vi "mislanius_time_add_all.vi"(0 "Select Product":string, 1 "Cluster":T2={"connection reference"=refnum, "Net Avai time (Min)"=0, "pLAN dATE datA"=[], "Data by plan date, shift, product"=[], "BreakDownd Data"=[], "Raw rejection Data"=[], "mislanius times shift 1"={"Lunch Time From"=timestamp(0 s since 1904-01-01), "Lunch Time To"=timestamp(0 s since 1904-01-01), "Tea Time From"=timestamp(0 s since 1904-01-01), "Tea Time To"=timestamp(0 s since 1904-01-01), "Clean Time From"=timestamp(0 s since 1904-01-01), "Clean Time To"=timestamp(0 s since 1904-01-01), "Meeting Time From"=timestamp(0 s since 1904-01-01), "Meeting Time To"=timestamp(0 s since 1904-01-01), "Dev/Other Time From"=timestamp(0 s since 1904-01-01), "Dev/Other Time To"=timestamp(0 s since 1904-01-01), "Meeting"=FALSE, "Dev/Other"=TRUE}, "mislanius times shift 2"={"Lunch Time From"=timestamp(0 s since 1904-01-01), "Lunch Time To"=timestamp(0 s since 1904-01-01), "Tea Time From"=timestamp(0 s since 1904-01-01), "Tea Time To"=timestamp(0 s since 1904-01-01), "Clean Time From"=timestamp(0 s since 1904-01-01), "Clean Time To"=timestamp(0 s since 1904-01-01), "Meeting Time From"=timestamp(0 s since 1904-01-01), "Meeting Time To"=timestamp(0 s since 1904-01-01), "Dev/Other Time From"=timestamp(0 s since 1904-01-01), "Dev/Other Time To"=timestamp(0 s since 1904-01-01), "Meeting"=FALSE, "Dev/Other"=TRUE}} {"mislanius times shift 2"."Lunch Time From" format="%<%.X %x>T"; "mislanius times shift 2"."Lunch Time To" format="%<%.X %x>T"; "mislanius times shift 2"."Tea Time From" format="%<%.X %x>T"; "mislanius times shift 2"."Tea Time To" format="%<%.X %x>T"; "mislanius times shift 2"."Clean Time From" format="%<%.X %x>T"; "mislanius times shift 2"."Clean Time To" format="%<%.X %x>T"; "mislanius times shift 2"."Meeting Time From" format="%<%.X %x>T"; "mislanius times shift 2"."Meeting Time To" format="%<%.X %x>T"; "mislanius times shift 2"."Dev/Other Time From" format="%<%.X %x>T"; "mislanius times shift 2"."Dev/Other Time To" format="%<%.X %x>T"; "mislanius times shift 1"."Lunch Time From" format="%<%.X %x>T"; "mislanius times shift 1"."Lunch Time To" format="%<%.X %x>T"; "mislanius times shift 1"."Tea Time From" format="%<%.X %x>T"; "mislanius times shift 1"."Tea Time To" format="%<%.X %x>T"; "mislanius times shift 1"."Clean Time From" format="%<%.X %x>T"; "mislanius times shift 1"."Clean Time To" format="%<%.X %x>T"; "mislanius times shift 1"."Meeting Time From" format="%<%.X %x>T"; "mislanius times shift 1"."Meeting Time To" format="%<%.X %x>T"; "mislanius times shift 1"."Dev/Other Time From" format="%<%.X %x>T"; "mislanius times shift 1"."Dev/Other Time To" format="%<%.X %x>T"}, 2 "error in (no error)":errorcluster, 3 "Date":timestamp, 8 "Shift":string(combo)="2") -> (6 "AT min":i32, 10 "Split DT time":u32[](array[numeric]), 12 "Only select product and date and shift data":string[][](array[string]), 15 "1st and last cycle time stamp":timestamp[](array[timestamp]), 16 "error out":errorcluster, 17 "Net Available Time":u32, 18 "output cluster":T1, 19 "Total mis time":i32)   [LabVIEW 2017]
uses:
  Controls/OE_screen_cluster.ctl
  <vilib>/addons/database/Connection.llb/Conn ObjectReference.ctl
  <userlib>/_OpenG.lib/array/array.llb/Remove Duplicates from 1D Array (String)__ogtk.vi
  <userlib>/_OpenG.lib/array/array.llb/Search 1D Array (String)__ogtk.vi
  <userlib>/_OpenG.lib/array/array.llb/Remove Duplicates from 1D Array (I32)__ogtk.vi
  <vilib>/addons/database/NI_Database_API.lvlib
panel:
  out "Array":string[](array[string])
  out "x-1 3":timestamp[](array[timestamp])
  out "Array 2":timestamp[](array[timestamp])
  out "indices of removed elements":i32[](array[numeric])
  out "Only rejected- select product and date and shift data":string[][](array[string])
  out "Parts per hour":i32
  out "Lunch time 3":i32
  out "tea time 3":i32
  out "clean time 3":i32
  out "meeting time 3":i32
  out "Dev/other time 3":i32
  out "Lunch time 2":i32
  out "tea time 2":i32
  out "clean time 2":i32
  out "meeting time 2":i32
  out "Dev/other time 2":i32
  out "Dev/other time":i32
  out "meeting time":i32
  out "clean time":i32
  out "tea time":i32
  out "Lunch time":i32
  out "In Range? 5":bool
  out "In Range? 4":bool
  out "In Range? 3":bool
  out "In Range? 2":bool
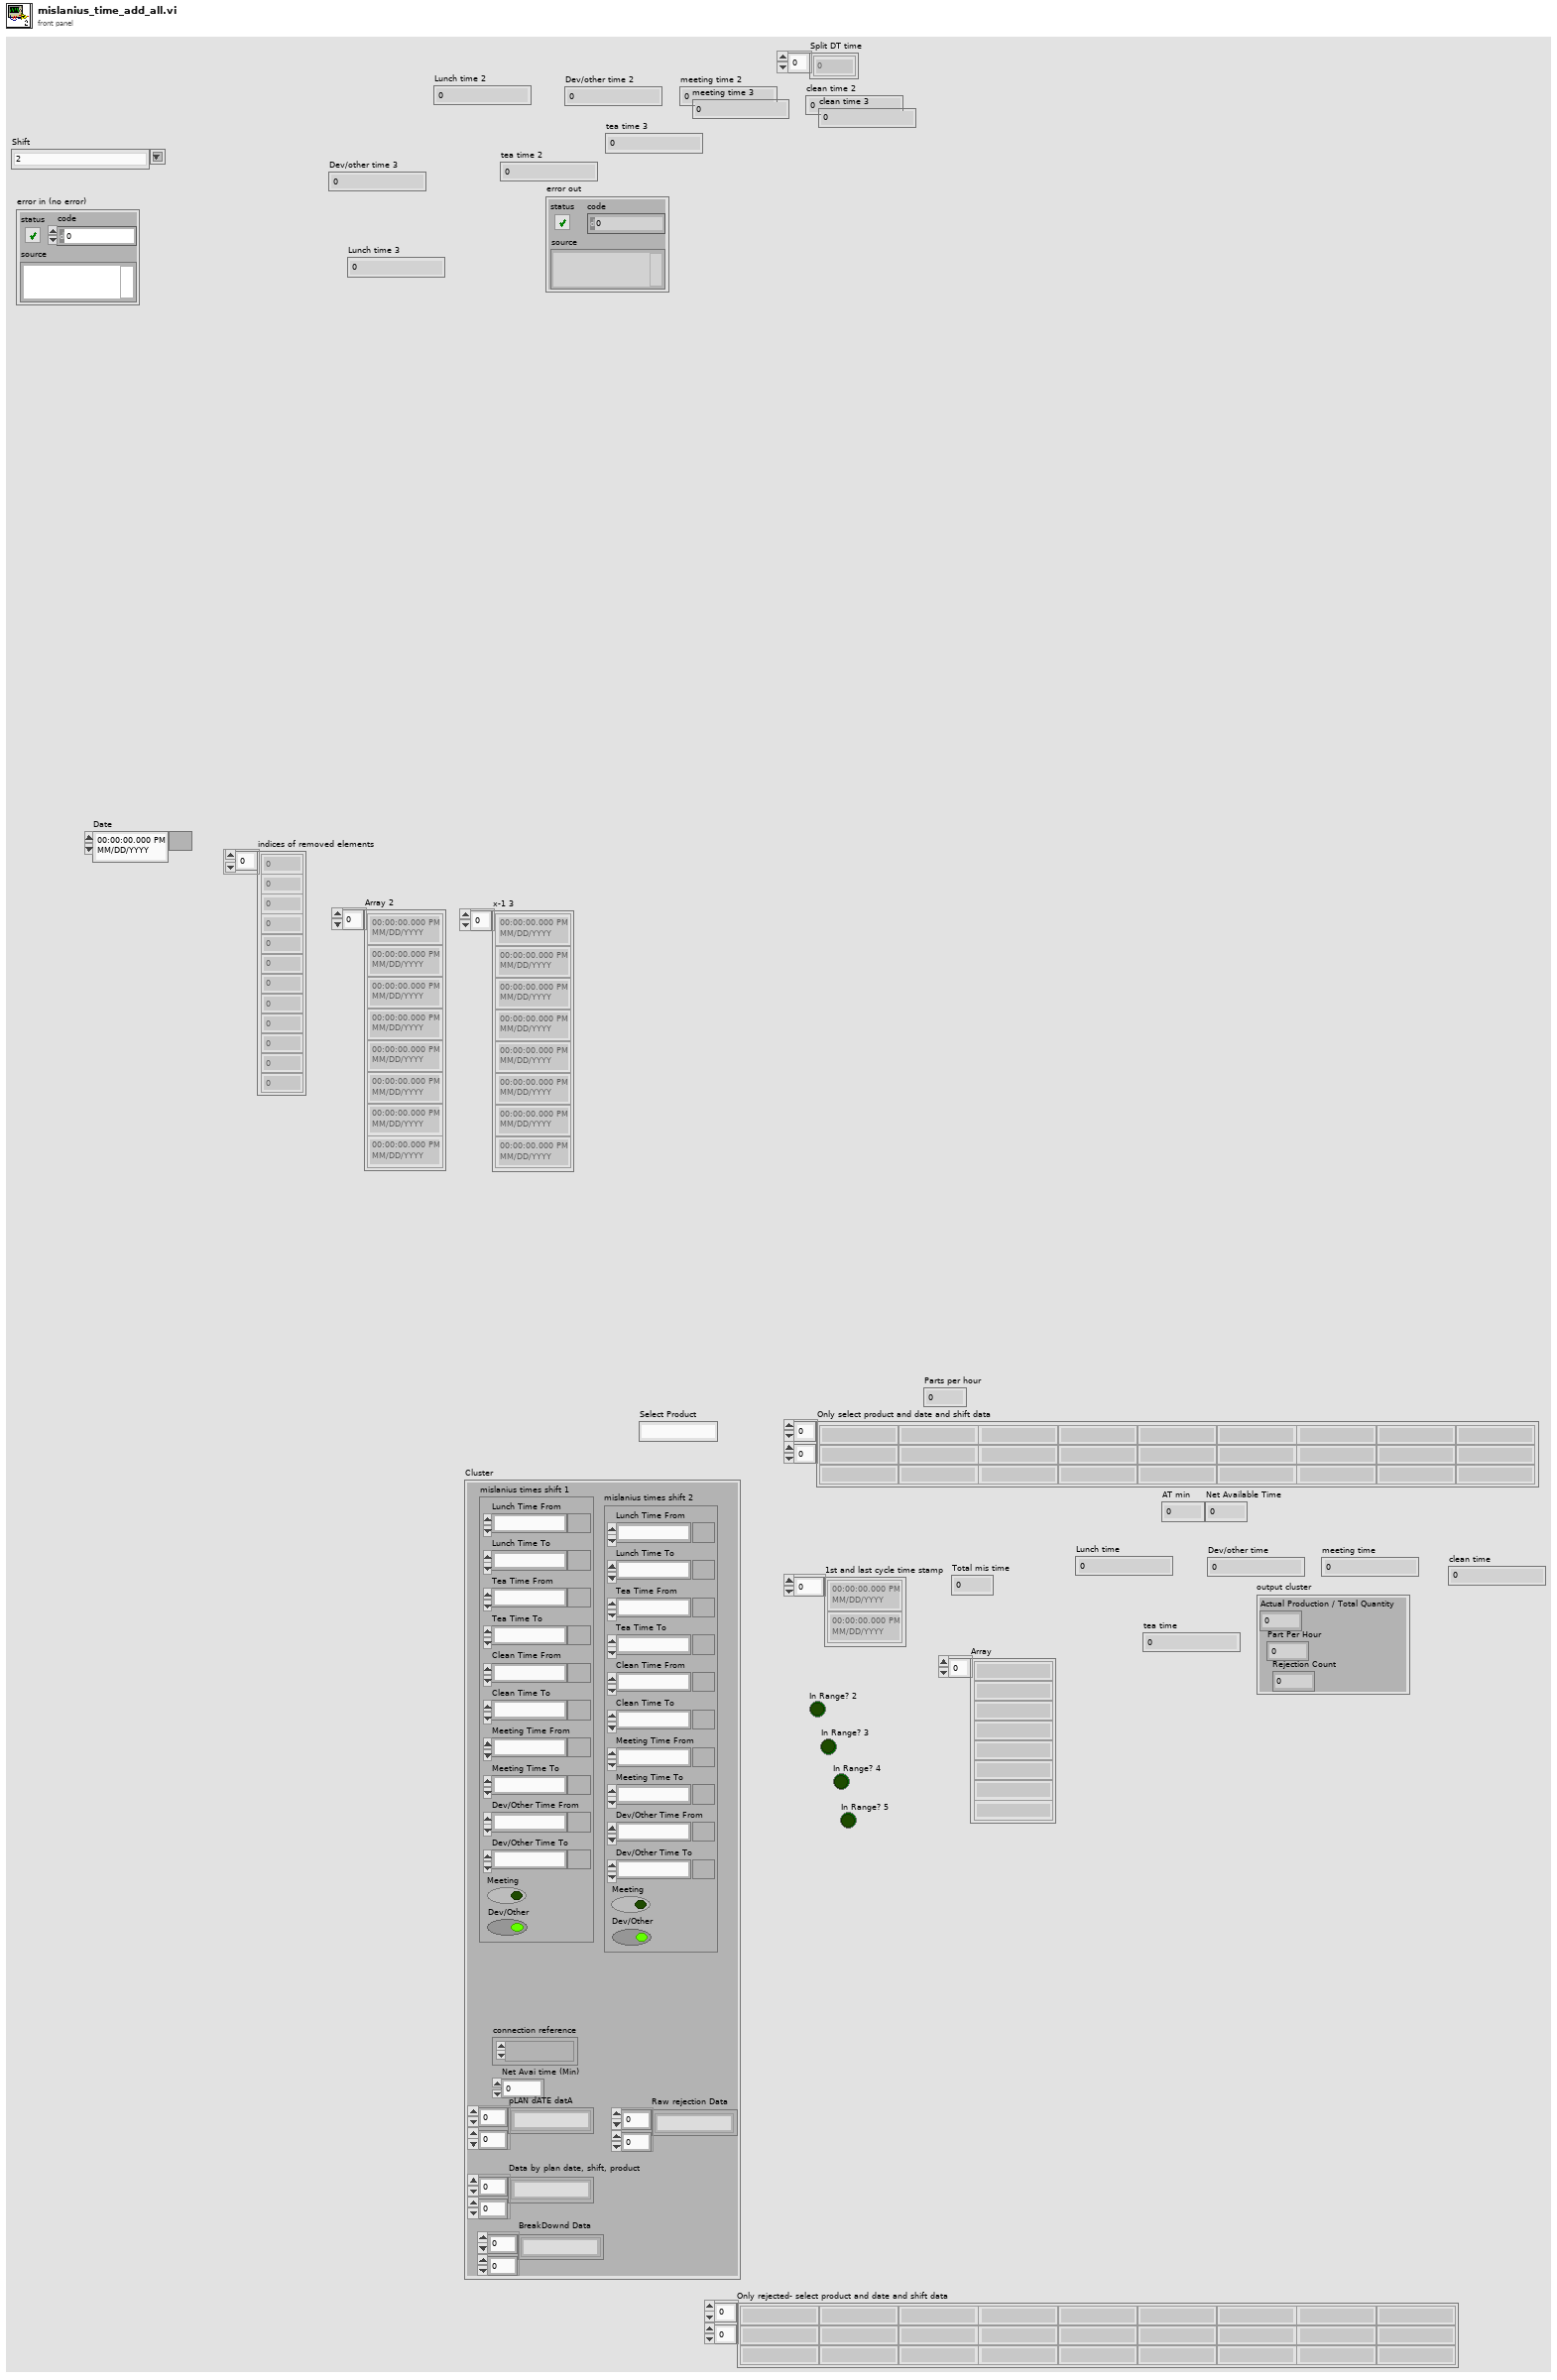
[diagram p1: front panel]
types:
  T1 = cluster{"Actual Production / Total Quantity":u32, "Part Per Hour":i16, "Rejection Count":u32}
  T2 = typedef "OE_screen_cluster.ctl" = cluster{"connection reference":T3, "Net Avai time (Min)":i32, "pLAN dATE datA":string[][], "Data by plan date, shift, product":string[][], "BreakDownd Data":string[][], "Raw rejection Data":string[][], "mislanius times shift 1":cluster{"Lunch Time From":timestamp, "Lunch Time To":timestamp, "Tea Time From":timestamp, "Tea Time To":timestamp, "Clean Time From":timestamp, "Clean Time To":timestamp, "Meeting Time From":timestamp, "Meeting Time To":timestamp, "Dev/Other Time From":timestamp, "Dev/Other Time To":timestamp, "Meeting":bool, "Dev/Other":bool}, "mislanius times shift 2":cluster{"Lunch Time From":timestamp, "Lunch Time To":timestamp, "Tea Time From":timestamp, "Tea Time To":timestamp, "Clean Time From":timestamp, "Clean Time To":timestamp, "Meeting Time From":timestamp, "Meeting Time To":timestamp, "Dev/Other Time From":timestamp, "Dev/Other Time To":timestamp, "Meeting":bool, "Dev/Other":bool}}
  T3 = typedef "NI_Database_API.lvlib/Conn ObjectReference.ctl" = refnum<k1>
  T4 = typedef "LVDateTimeRec.ctl" = cluster{"fractional second":dbl, "second":i32, "minute":i32, "hour":i32, "day of month":i32, "month":i32, "year":i32, "day of week":i32, "day of year":i32, "DST":i32}
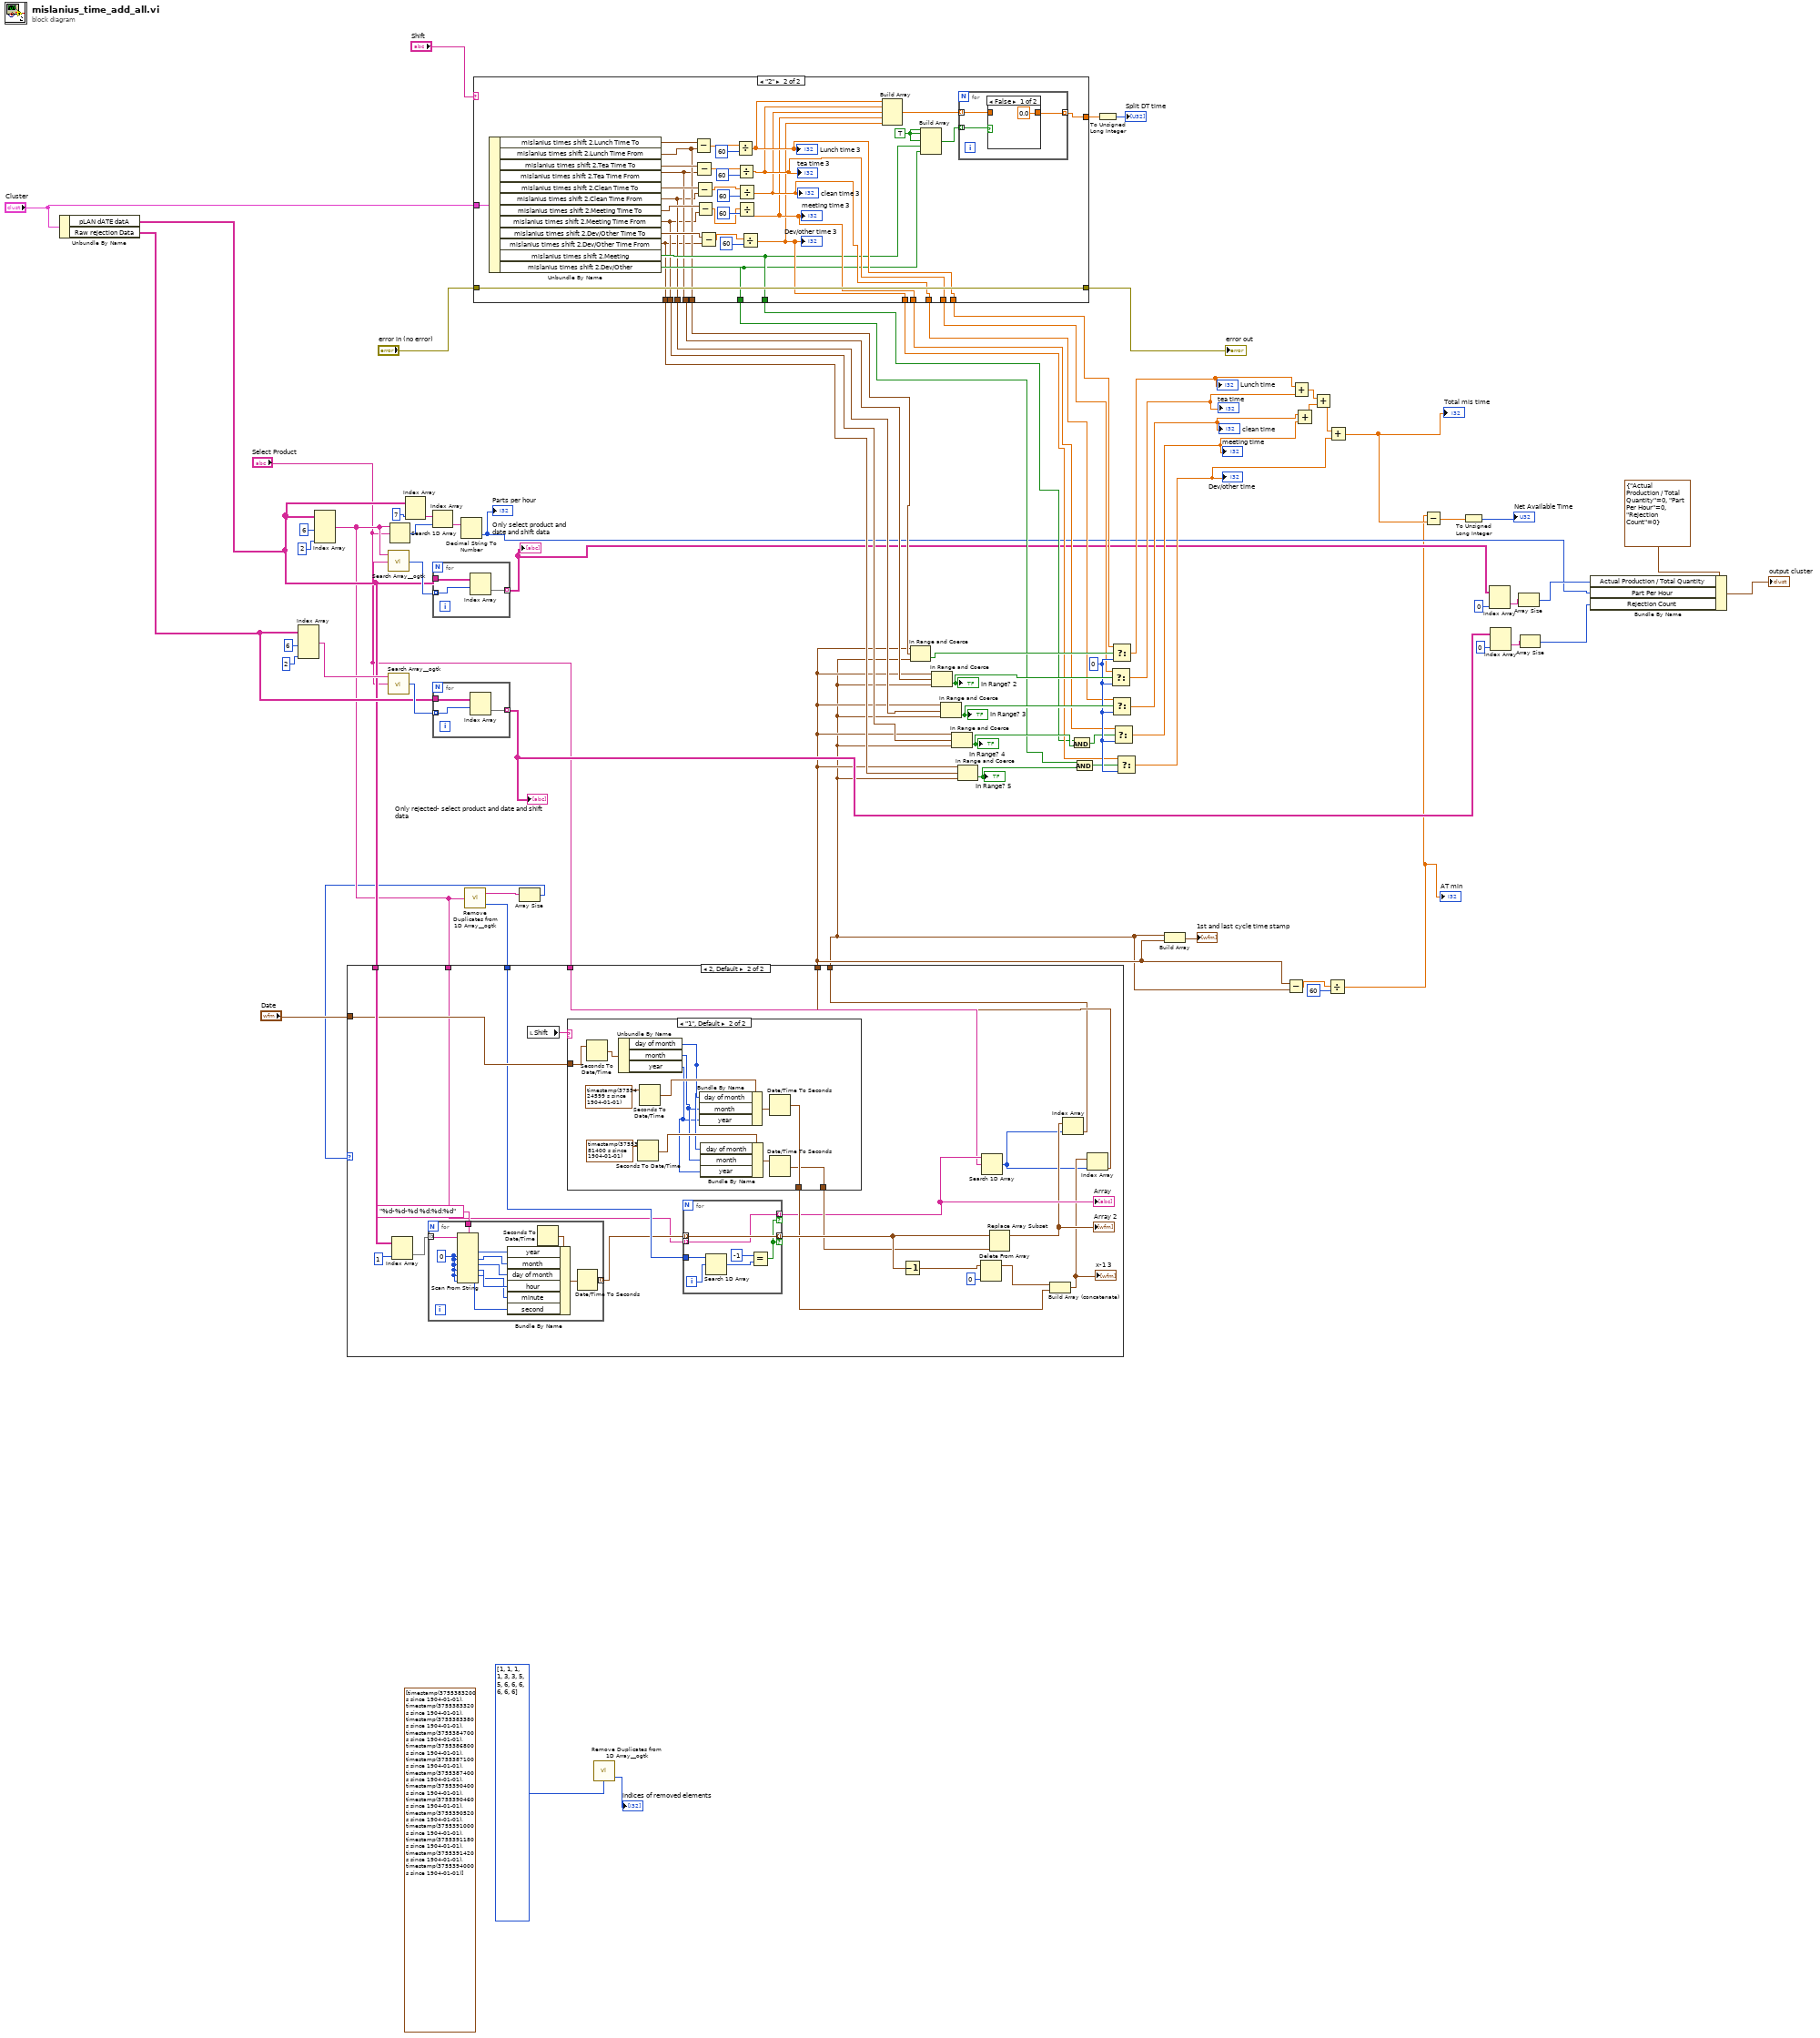
[diagram p0: block diagram]
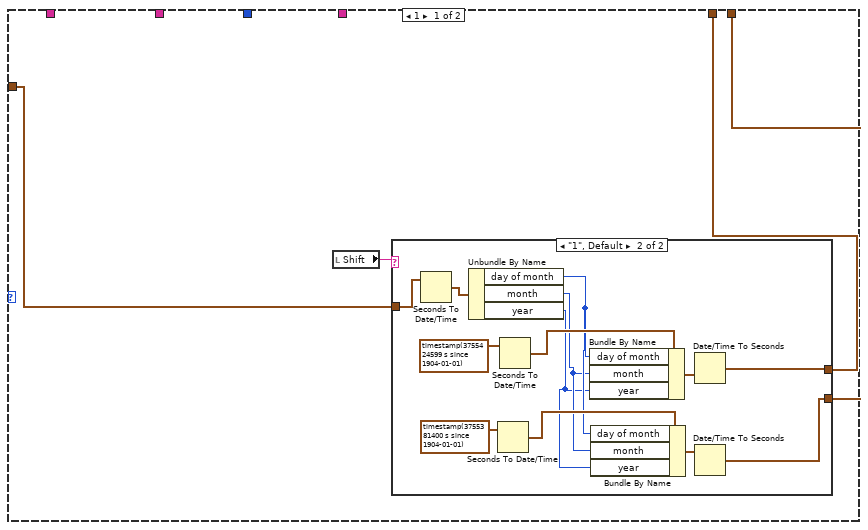
[diagram p2: hidden frame]
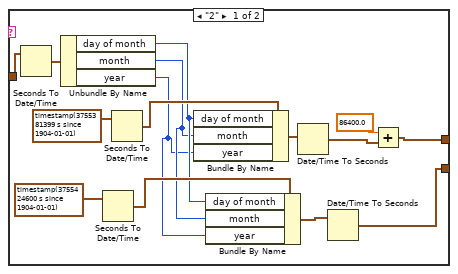
[diagram p3: hidden frame]
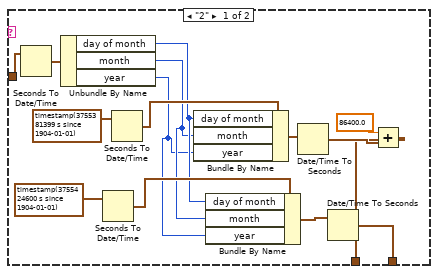
[diagram p4: hidden frame]
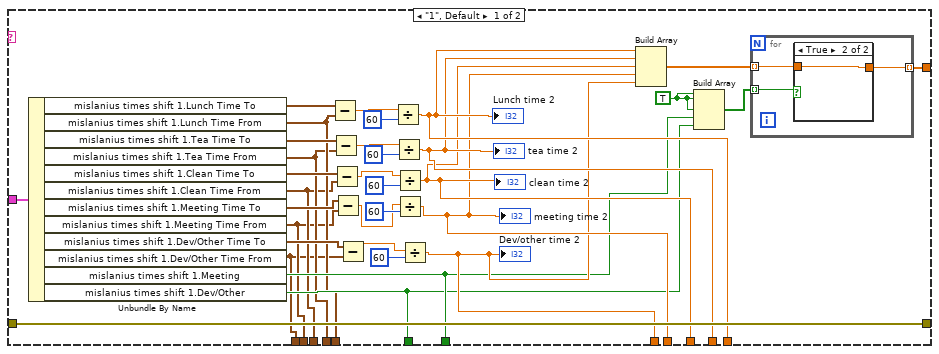
[diagram p5: hidden frame]
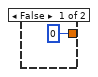
[diagram p6: hidden frame]
diagram:
  (unwired) timestamp[] [timestamp(3755383200 s since 1904-01-01), timestamp(3755383320 s since 1904-01-01), timestamp(3755383380 s since 1904-01-01), timestamp(3755384700 s since 1904-01-01), timestamp(3755386800 s since 1904-01-01), timestamp(3755387100 s since 1904-01-01), timestamp(3755387400 s since 1904-01-01), timestamp(3755390400 s since 1904-01-01), timestamp(3755390460 s since 1904-01-01), timestamp(3755390520 s since 1904-01-01), timestamp(3755391000 s since 1904-01-01), timestamp(3755391180 s since 1904-01-01), timestamp(3755391420 s since 1904-01-01), timestamp(3755394000 s since 1904-01-01)]
  w66 = 0
  n1 = Unbundle By Name("Cluster") -> ("pLAN dATE datA"=w14:string[][], "Raw rejection Data"=w27:string[][])
  n2 = Index Array(array=w27, index (col) #1=6 ("disabled index (col)"), index (col) #2=2 ("disabled index (col)")) -> (element #1=w50:string[])  [unwired: 2 in, 1 out]
  n3 = Index Array(array=w14, index (col) #1=6 ("disabled index (col)"), index (col) #2=2 ("disabled index (col)")) -> (element #1=w9:string[])  [unwired: 2 in, 1 out]
  n4 = call-poly <userlib>:"Search Array__ogtk.vi"("Array"=w9, "Element Data"="Select Product") -> ("Indices of Elements"=w75:i32[])  [unwired: 7 in]
  n5 = call-poly <userlib>:"Search Array__ogtk.vi"("Array"=w50, "Element Data"="Select Product") -> ("Indices of Elements"=w51:i32[])  [unwired: 7 in]
  n6 = Search 1D Array(1D array=w9, element="Select Product") -> (index of element=w73:i32)  [unwired: 1 in]
  n7 = Index Array(array=w14, index (col)=7 ("disabled index (col)")) -> (element=w72:string[])  [unwired: 1 in]
  n8 = Index Array(array=w72, index=w73) -> (element=w74:string)
  n9 = for {
    tunnel: w14 -> [w78]
    tunnel: w75 -> [w77] mode=indexing
    tunnel: [w76] -> w22 mode=indexing
    n10 = Index Array(array=w78, index (row)=w77) -> (element=w76:string[])  [unwired: 1 in]
  }
  "Only select product and date and shift data" <- w22
  n11 = for {
    tunnel: w27 -> [w81]
    tunnel: w51 -> [w80] mode=indexing
    tunnel: [w79] -> w16 mode=indexing
    n12 = Index Array(array=w81, index (row)=w80) -> (element=w79:string[])  [unwired: 1 in]
  }
  "Only rejected- select product and date and shift data" <- w16
  n13 = Decimal String To Number(string=w74) -> (number=w20:i32)  [unwired: 2 in, 1 out]
  "Parts per hour" <- w20
  n14 = call-poly <userlib>:"Remove Duplicates from 1D Array__ogtk.vi"("Input Array"=w9) -> ("Output Array"=w15:string[], "indices of removed elements"=w11:i32[])
  n15 = case shown="\"2\"" "Shift" {
    tunnel: "Cluster" -> [w99 w137]
    tunnel: [w98 w136] -> w48
    tunnel: "error in (no error)" -> [w98 w136]
    tunnel: [w94 w133] -> w46
    tunnel: [w93 w131] -> w42
    tunnel: [w92 w130] -> w41
    tunnel: [w91 w129] -> w40
    tunnel: [w90 w128] -> w39
    tunnel: [w89 w127] -> w38
    tunnel: [w88 w126] -> w37
    tunnel: [w87 w125] -> w36
    tunnel: [w86 w124] -> w33
    tunnel: [w85 w123] -> w32
    tunnel: [w84 w122] -> w31
    tunnel: [w83 w121] -> w30
    tunnel: [w82 w120] -> w29
    frame "1", Default {
      w96 = TRUE
      n16 = Unbundle By Name(w99) -> ("mislanius times shift 1.Lunch Time To"=w112:timestamp, "mislanius times shift 1.Lunch Time From"=w86:timestamp, "mislanius times shift 1.Tea Time To"=w111:timestamp, "mislanius times shift 1.Tea Time From"=w85:timestamp, "mislanius times shift 1.Clean Time To"=w107:timestamp, "mislanius times shift 1.Clean Time From"=w84:timestamp, "mislanius times shift 1.Meeting Time To"=w104:timestamp, "mislanius times shift 1.Meeting Time From"=w83:timestamp, "mislanius times shift 1.Dev/Other Time To"=w100:timestamp, "mislanius times shift 1.Dev/Other Time From"=w82:timestamp, "mislanius times shift 1.Meeting"=w88:bool, "mislanius times shift 1.Dev/Other"=w87:bool)
      n17 = Subtract(x=w112, y=w86) -> (x-y=w114:dbl)
      n18 = Subtract(x=w111, y=w85) -> (x-y=w109:dbl)
      n19 = Subtract(x=w107, y=w84) -> (x-y=w105:dbl)
      n20 = Subtract(x=w104, y=w83) -> (x-y=w103:dbl)
      n21 = Subtract(x=w100, y=w82) -> (x-y=w102:dbl)
      n22 = Divide(x=w114, y=60) -> (x/y=w93:dbl)
      "Lunch time 2" <- w93
      n23 = Divide(x=w109, y=60) -> (x/y=w92:dbl)
      "tea time 2" <- w92
      n24 = Divide(x=w105, y=60) -> (x/y=w91:dbl)
      "clean time 2" <- w91
      n25 = Divide(x=w103, y=60) -> (x/y=w90:dbl)
      "meeting time 2" <- w90
      n26 = Divide(x=w102, y=60) -> (x/y=w89:dbl)
      "Dev/other time 2" <- w89
      n27 = Build Array(w93, w92, w91, w90, w89) -> (w97:dbl[])
      n28 = Build Array(w96, w96, w96, w88, w87) -> (w95:bool[])
      n29 = for {
        tunnel: w97 -> [w115] mode=indexing
        tunnel: w95 -> [w117] mode=indexing
        tunnel: [w116] -> w94 mode=indexing
        n30 = case shown="True" w117 {
          tunnel: [0 w119] -> w116
          tunnel: w115 -> [_ w119]
          frame False {
          }
          frame True {
          }
        }
      }
    }
    frame "2" {
      w134 = TRUE
      n31 = Unbundle By Name(w137) -> ("mislanius times shift 2.Lunch Time To"=w150:timestamp, "mislanius times shift 2.Lunch Time From"=w124:timestamp, "mislanius times shift 2.Tea Time To"=w149:timestamp, "mislanius times shift 2.Tea Time From"=w123:timestamp, "mislanius times shift 2.Clean Time To"=w145:timestamp, "mislanius times shift 2.Clean Time From"=w122:timestamp, "mislanius times shift 2.Meeting Time To"=w142:timestamp, "mislanius times shift 2.Meeting Time From"=w121:timestamp, "mislanius times shift 2.Dev/Other Time To"=w138:timestamp, "mislanius times shift 2.Dev/Other Time From"=w120:timestamp, "mislanius times shift 2.Meeting"=w126:bool, "mislanius times shift 2.Dev/Other"=w125:bool)
      n32 = Subtract(x=w150, y=w124) -> (x-y=w152:dbl)
      n33 = Subtract(x=w149, y=w123) -> (x-y=w147:dbl)
      n34 = Subtract(x=w145, y=w122) -> (x-y=w143:dbl)
      n35 = Subtract(x=w142, y=w121) -> (x-y=w141:dbl)
      n36 = Subtract(x=w138, y=w120) -> (x-y=w140:dbl)
      n37 = Divide(x=w152, y=60) -> (x/y=w131:dbl)
      "Lunch time 3" <- w131
      n38 = Divide(x=w147, y=60) -> (x/y=w130:dbl)
      "tea time 3" <- w130
      n39 = Divide(x=w143, y=60) -> (x/y=w129:dbl)
      "clean time 3" <- w129
      n40 = Divide(x=w141, y=60) -> (x/y=w128:dbl)
      "meeting time 3" <- w128
      n41 = Divide(x=w140, y=60) -> (x/y=w127:dbl)
      "Dev/other time 3" <- w127
      n42 = Build Array(w131, w130, w129, w128, w127) -> (w132:dbl[])
      n43 = Build Array(w134, w134, w134, w126, w125) -> (w135:bool[])
      n44 = for {
        tunnel: w132 -> [w153] mode=indexing
        tunnel: w135 -> [w155] mode=indexing
        tunnel: [w154] -> w133 mode=indexing
        n45 = case shown="False" w155 {
          tunnel: [0.0 w157] -> w154
          tunnel: w153 -> [_ w157]
          frame False {
          }
          frame True {
          }
        }
      }
    }
  }
  "error out" <- w48
  n46 = Array Size(array=w15) -> (size(s)=w1:i32)
  n47 = case shown="2, Default" w1 {
    tunnel: w14 -> [_ w210]
    tunnel: "Date" -> [w160 w203]
    tunnel: w11 -> [_ w201]
    tunnel: w9 -> [_ w197]
    tunnel: "Select Product" -> [_ w195]
    tunnel: [w159 w191] -> w4
    tunnel: [w158 w190] -> w3
    frame 1 {
      n48 = local read "Shift"() -> (w161:string)
      n49 = case shown="\"1\", Default" w161 {
        tunnel: [w169 w180] -> w158
        tunnel: [w165 w185] -> w159
        tunnel: w160 -> [w168 w182]
        frame "2" {
          n50 = Seconds To Date/Time(time stamp (now)=w168) -> (date time rec=w174:T4)  [unwired: 1 in]
          n51 = Unbundle By Name(w174) -> ("day of month"=w164:i32, "month"=w163:i32, "year"=w162:i32)
          n52 = Seconds To Date/Time(time stamp (now)=timestamp(3755424600 s since 1904-01-01)) -> (date time rec=w171:T4)  [unwired: 1 in]
          n53 = Seconds To Date/Time(time stamp (now)=timestamp(3755381399 s since 1904-01-01)) -> (date time rec=w175:T4)  [unwired: 1 in]
          n54 = Bundle By Name(cluster=w175, "day of month"=w164, "month"=w163, "year"=w162) -> (w176:T4)
          n55 = Bundle By Name(cluster=w171, "day of month"=w164, "month"=w163, "year"=w162) -> (w172:T4)
          n56 = Date/Time To Seconds(2:w176) -> (0:w166:timestamp)  [unwired: 1 in]
          n57 = Date/Time To Seconds(2:w172) -> (0:w169:timestamp)  [unwired: 1 in]
          n58 = Add(x=86400.0 ("x-y 2"), y=w166) -> (x+y=w165:timestamp)
        }
        frame "1", Default {
          n59 = Seconds To Date/Time(time stamp (now)=w182) -> (date time rec=w187:T4)  [unwired: 1 in]
          n60 = Unbundle By Name(w187) -> ("day of month"=w179:i32, "month"=w178:i32, "year"=w177:i32)
          n61 = Seconds To Date/Time(time stamp (now)=timestamp(3755381400 s since 1904-01-01)) -> (date time rec=w184:T4)  [unwired: 1 in]
          n62 = Seconds To Date/Time(time stamp (now)=timestamp(3755424599 s since 1904-01-01)) -> (date time rec=w188:T4)  [unwired: 1 in]
          n63 = Bundle By Name(cluster=w188, "day of month"=w179, "month"=w178, "year"=w177) -> (w189:T4)
          n64 = Bundle By Name(cluster=w184, "day of month"=w179, "month"=w178, "year"=w177) -> (w181:T4)
          n65 = Date/Time To Seconds(2:w189) -> (0:w185:timestamp)  [unwired: 1 in]
          n66 = Date/Time To Seconds(2:w181) -> (0:w180:timestamp)  [unwired: 1 in]
        }
      }
    }
    frame 2, Default {
      n67 = Index Array(array=w210, index (col)=1 ("index (row)")) -> (element=w198:string[])  [unwired: 1 in]
      n68 = for {
        tunnel: "%d-%d-%d %d:%d:%d" ("time format string (%c)") -> [w223]
        tunnel: [w213] -> w199 mode=indexing
        tunnel: w198 -> [w212] mode=indexing
        w215 = 0
        n69 = Scan From String(format string=w223, input string=w212, default 1=w215, default 2=w215, default 3=w215, default 4=w215, default 5=w215, default 6=w215) -> (output 1=w221:i32, output 2=w220:i32, output 3=w219:i32, output 4=w218:i32, output 5=w217:i32, output 6=w216:i32)  [unwired: 2 in, 3 out]
        n70 = Seconds To Date/Time() -> (date time rec=w222:T4)  [unwired: 2 in]
        n71 = Bundle By Name(cluster=w222, "year"=w221, "month"=w220, "day of month"=w219, "hour"=w218, "minute"=w217, "second"=w216) -> (w214:T4)
        n72 = Date/Time To Seconds(2:w214) -> (0:w213:timestamp)  [unwired: 1 in]
      }
      n73 = local read "Shift"() -> (w202:string)
      n74 = case shown="\"1\", Default" w202 {
        tunnel: [w231 w242] -> w205
        tunnel: [w227 w247] -> w204
        tunnel: w203 -> [w230 w244]
        frame "2" {
          n75 = Seconds To Date/Time(time stamp (now)=w230) -> (date time rec=w236:T4)  [unwired: 1 in]
          n76 = Unbundle By Name(w236) -> ("day of month"=w226:i32, "month"=w225:i32, "year"=w224:i32)
          n77 = Seconds To Date/Time(time stamp (now)=timestamp(3755424600 s since 1904-01-01)) -> (date time rec=w233:T4)  [unwired: 1 in]
          n78 = Seconds To Date/Time(time stamp (now)=timestamp(3755381399 s since 1904-01-01)) -> (date time rec=w237:T4)  [unwired: 1 in]
          n79 = Bundle By Name(cluster=w237, "day of month"=w226, "month"=w225, "year"=w224) -> (w238:T4)
          n80 = Bundle By Name(cluster=w233, "day of month"=w226, "month"=w225, "year"=w224) -> (w234:T4)
          n81 = Date/Time To Seconds(2:w238) -> (0:w228:timestamp)  [unwired: 1 in]
          n82 = Date/Time To Seconds(2:w234) -> (0:w231:timestamp)  [unwired: 1 in]
          n83 = Add(x=86400.0 ("x-y 2"), y=w228) -> (x+y=w227:timestamp)
        }
        frame "1", Default {
          n84 = Seconds To Date/Time(time stamp (now)=w244) -> (date time rec=w249:T4)  [unwired: 1 in]
          n85 = Unbundle By Name(w249) -> ("day of month"=w241:i32, "month"=w240:i32, "year"=w239:i32)
          n86 = Seconds To Date/Time(time stamp (now)=timestamp(3755381400 s since 1904-01-01)) -> (date time rec=w246:T4)  [unwired: 1 in]
          n87 = Seconds To Date/Time(time stamp (now)=timestamp(3755424599 s since 1904-01-01)) -> (date time rec=w250:T4)  [unwired: 1 in]
          n88 = Bundle By Name(cluster=w250, "day of month"=w241, "month"=w240, "year"=w239) -> (w251:T4)
          n89 = Bundle By Name(cluster=w246, "day of month"=w241, "month"=w240, "year"=w239) -> (w243:T4)
          n90 = Date/Time To Seconds(2:w251) -> (0:w247:timestamp)  [unwired: 1 in]
          n91 = Date/Time To Seconds(2:w243) -> (0:w242:timestamp)  [unwired: 1 in]
        }
      }
      n92 = for {
        tunnel: w199 -> [w254] mode=indexing
        tunnel: w201 -> [w257]
        tunnel: [w254] -> w209 mode=indexing if=w252
        tunnel: w197 -> [w253] mode=indexing
        tunnel: [w253] -> w196 mode=indexing if=w252
        i -> [w258]
        n93 = Search 1D Array(1D array=w257, element=w258) -> (index of element=w256:i32)  [unwired: 1 in]
        n94 = Equal?(x=-1, y=w256) -> (x = y?=w252:bool)
      }
      "Array" <- w196
      n95 = Decrement(x=w209) -> (x-1=w207:timestamp[])
      n96 = Delete From Array(array=w207, index=0) -> (array with subset deleted=w206:timestamp[])  [unwired: 1 in, 1 out]
      n97 = Search 1D Array(1D array=w196, element=w195) -> (index of element=w192:i32)  [unwired: 1 in]
      n98 = Replace Array Subset(array=w209, new element=w205) -> (w194:timestamp[])  [unwired: 1 in]
      "Array 2" <- w194
      n99 = Build Array (concatenate)(w206, w204) -> (w193:timestamp[])
      "x-1 3" <- w193
      n100 = Index Array(array=w194, index=w192) -> (element=w190:timestamp)
      n101 = Index Array(array=w193, index=w192) -> (element=w191:timestamp)
    }
  }
  n102 = call-poly <userlib>:"Remove Duplicates from 1D Array__ogtk.vi"("Input Array"=i32[] [1, 1, 1, 1, 3, 3, 5, 5, 6, 6, 6, 6, 6, 6]) -> ("indices of removed elements"=→"indices of removed elements":i32[])  [unwired: 1 out]
  n103 = In Range and Coerce(upper limit=w4, x=w33, lower limit=w3) -> (In Range?=w69:bool)  [unwired: 1 out]
  n104 = In Range and Coerce(upper limit=w4, x=w32, lower limit=w3) -> (In Range?=w67:bool)  [unwired: 1 out]
  "In Range? 2" <- w67
  n105 = In Range and Coerce(upper limit=w4, x=w31, lower limit=w3) -> (In Range?=w68:bool)  [unwired: 1 out]
  "In Range? 3" <- w68
  n106 = In Range and Coerce(upper limit=w4, x=w30, lower limit=w3) -> (In Range?=w59:bool)  [unwired: 1 out]
  "In Range? 4" <- w59
  n107 = In Range and Coerce(upper limit=w4, x=w29, lower limit=w3) -> (In Range?=w35:bool)  [unwired: 1 out]
  "In Range? 5" <- w35
  n108 = And(x=w37, y=w59) -> (x .and. y?=w58:bool)
  n109 = And(x=w36, y=w35) -> (x .and. y?=w34:bool)
  n110 = To Unsigned Long Integer(number=w46) -> (unsigned 32bit integer=→"Split DT time":u32[])
  n111 = Select(t=w41, s=w67, f=w66) -> (s? t:f=w61:dbl)
  "tea time" <- w61
  n112 = Select(t=w42, s=w69, f=w66) -> (s? t:f=w62:dbl)
  "Lunch time" <- w62
  n113 = Select(t=w40, s=w68, f=w66) -> (s? t:f=w60:dbl)
  "clean time" <- w60
  n114 = Select(t=w39, s=w58, f=w66) -> (s? t:f=w44:dbl)
  "meeting time" <- w44
  n115 = Select(t=w38, s=w34, f=w66) -> (s? t:f=w43:dbl)
  "Dev/other time" <- w43
  n116 = Build Array(w3, w4) -> (→"1st and last cycle time stamp":timestamp[])
  n117 = Subtract(x=w4, y=w3) -> (x-y=w5:dbl)
  n118 = Add(x=w62, y=w61) -> (x+y=w65:dbl)
  n119 = Add(x=w60, y=w44) -> (x+y=w64:dbl)
  n120 = Add(x=w65, y=w64) -> (x+y=w63:dbl)
  n121 = Divide(x=w5, y=60) -> (x/y=w2:dbl)
  "AT min" <- w2
  n122 = Add(x=w63, y=w43) -> (x+y=w56:dbl)
  "Total mis time" <- w56
  n123 = Subtract(x=w2, y=w56) -> (x-y=w55:dbl)
  n124 = To Unsigned Long Integer(number=w55) -> (unsigned 32bit integer=→"Net Available Time":u32)
  n125 = Index Array(array=w22, index (col)=0 ("disabled index (col)")) -> (element=w26:string[])  [unwired: 1 in]
  n126 = Index Array(array=w16, index (col)=0 ("disabled index (col)")) -> (element=w18:string[])  [unwired: 1 in]
  n127 = Array Size(array=w26) -> (size(s)=w23:i32)
  n128 = Array Size(array=w18) -> (size(s)=w17:i32)
  n129 = Bundle By Name(cluster=T1 {"Actual Production / Total Quantity"=0, "Part Per Hour"=0, "Rejection Count"=0}, "Actual Production / Total Quantity"=w23, "Part Per Hour"=w20, "Rejection Count"=w17) -> (→"output cluster":T1)
